vi "DMM_readout.vi"() -> ()   [LabVIEW 2009]
panel:
  out "Thermometer":dbl(slide) scale=0.0..400.0
  out "Numeric 2":i32
  in  "Samples Per Second 4":dbl=15.0
  out "CCS Resistance":dynamicdata(graph)
  out "Temperature":dbl
  out "Measurement taken":bool
  in  "stop":bool
  out "Heartbeat":bool
  in  "stop 2":bool
  out "DC coupled AC volts":string
  out "Resistance":string
  out "DC volts Chart":dbl(graph)
  out "DC volts":string
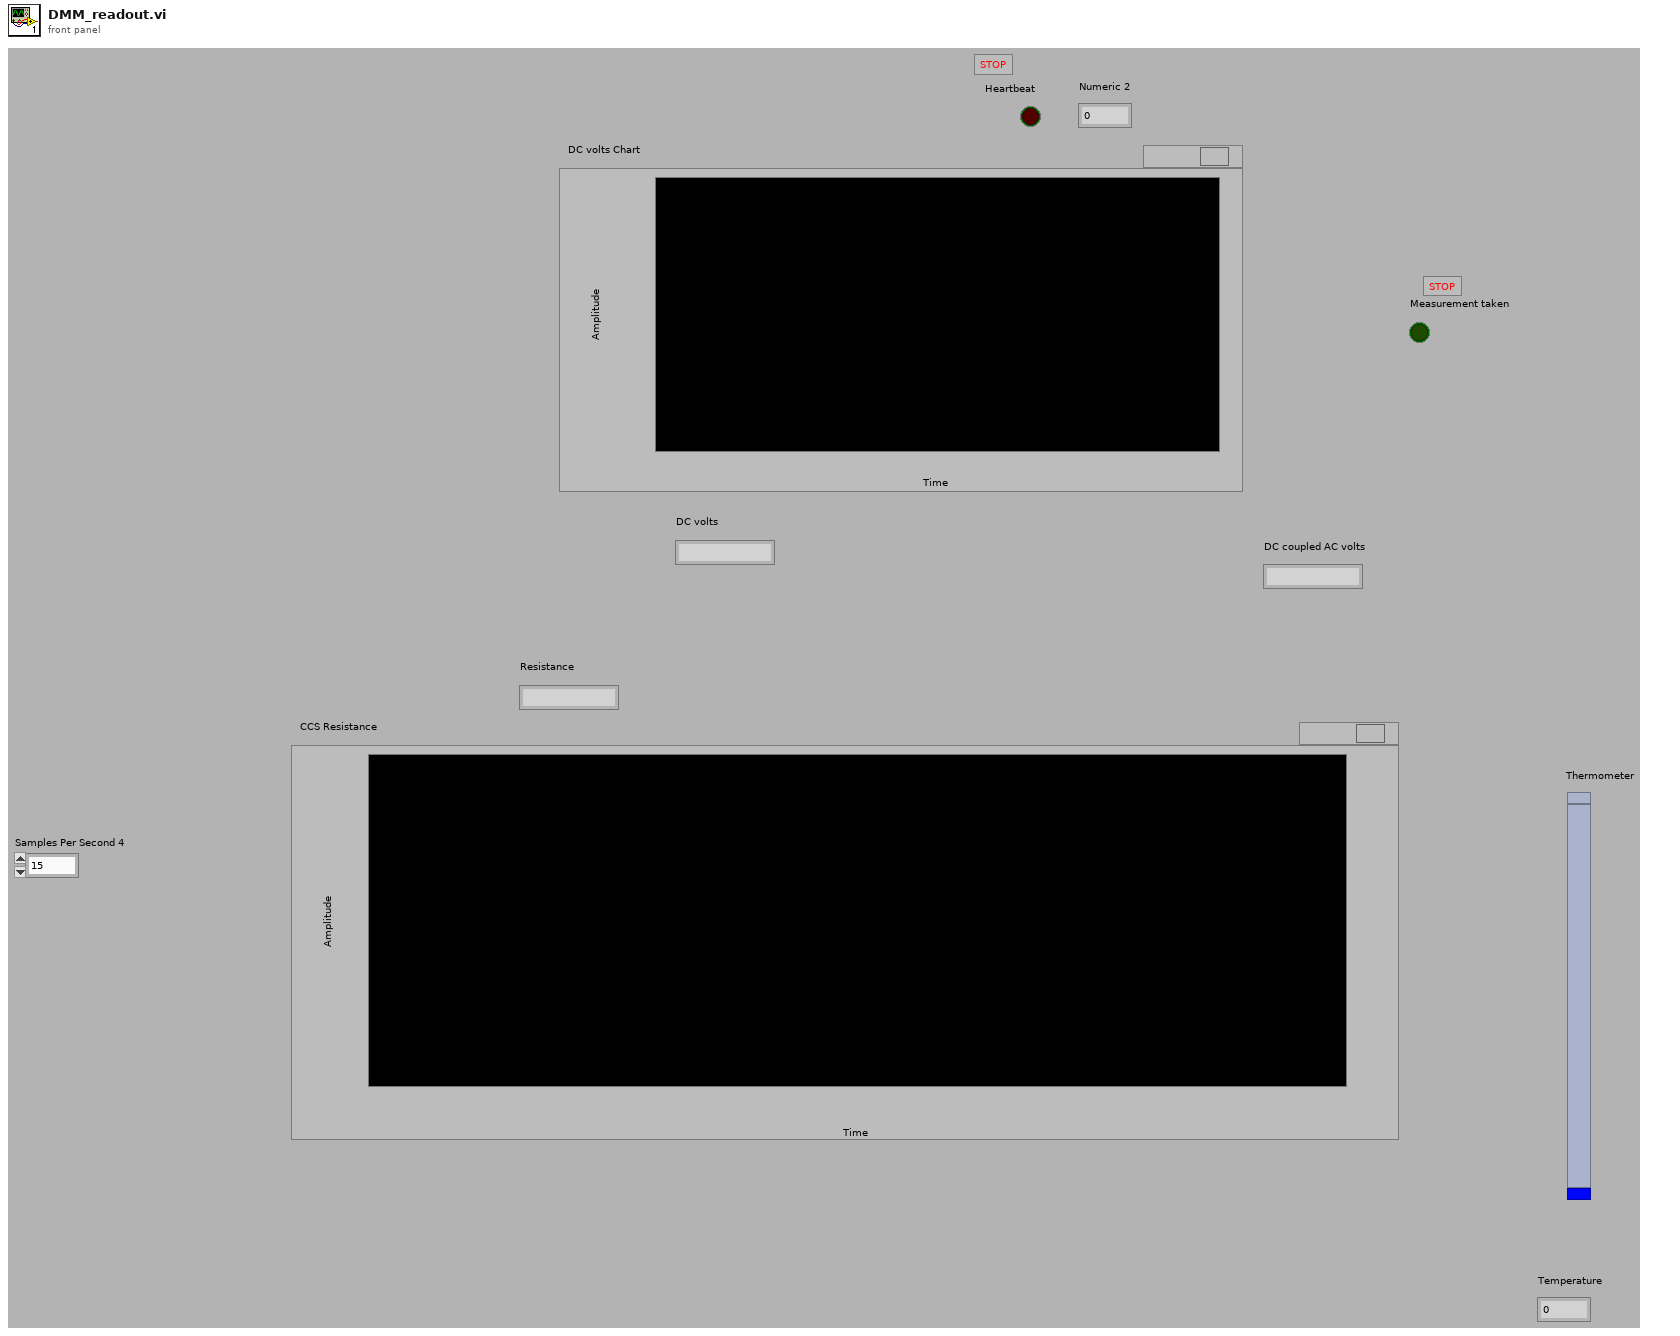
[diagram p1: front panel]
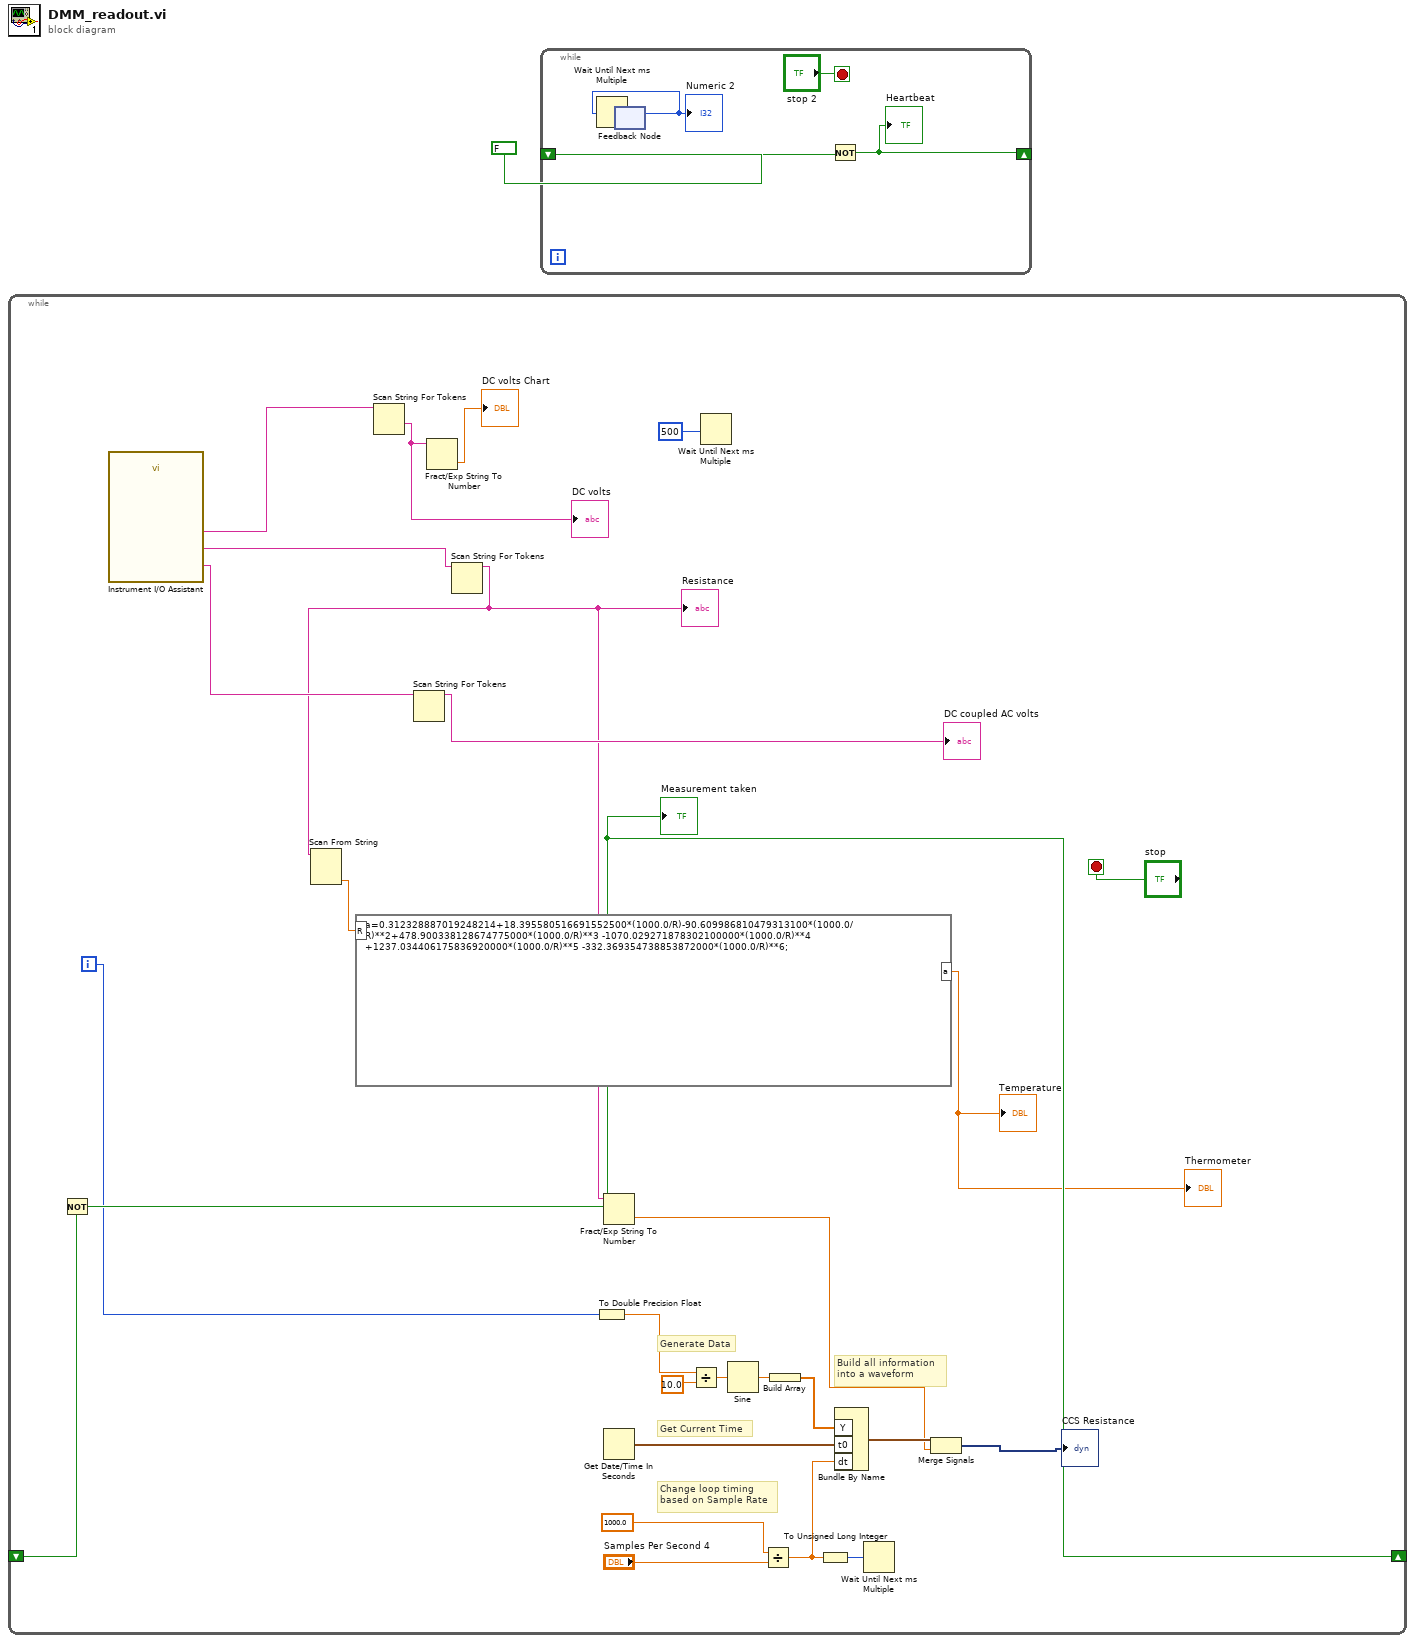
[diagram p0: block diagram]
diagram:
  n1 = while {
    shift-right: [w25] -> _
    shift-left: _ -> [w26]
    i -> [w5]
    stop <- "stop" stop-if-true
    # "Build all information\ninto a waveform"
    # "Change loop timing\nbased on Sample Rate"
    # "Get Current Time"
    # "Generate Data"
    n2 = Not(x=w26) -> (.not. x?=w25:bool)
    "Measurement taken" <- w25
    n3 = call "Instrument I/O Assistant"() -> ("DC coupled AC volts"=w20:string, "Resistance"=w18:string, "DC volts"=w23:string)  [unwired: 24 in, 1 out]
    n4 = Scan String For Tokens(9:w23) -> (1:w21:string)  [unwired: 5 in, 3 out]
    "DC volts" <- w21
    n5 = Scan String For Tokens(9:w20) -> (3:→"DC coupled AC volts":string)  [unwired: 5 in, 3 out]
    n6 = Fract/Exp String To Number(string=w21) -> (number=→"DC volts Chart":dbl)  [unwired: 3 in, 1 out]
    n7 = Scan String For Tokens(9:w18) -> (3:w17:string)  [unwired: 5 in, 3 out]
    "Resistance" <- w17
    n8 = Scan From String(input string=w17) -> (output 1=w22:dbl)  [unwired: 4 in, 3 out]
    n9 = formula code="a=0.312328887019248214+18.395580516691552500*(1000.0/R)-90.609986810479313100*(1000.0/R)**2+478.900338128674775000*(1000.0/R)**3 -1070.029271878302100000*(1000.0/R)**4 +1237.034406175836920000*(1000.0/R)**5 -332.369354738853872000*(1000.0/R)**6;"("R"=w22) -> ("a"=→"Temperature" →"Thermometer":dbl)
    n10 = To Double Precision Float(number=w5) -> (double precision float=w10:dbl)
    n11 = Fract/Exp String To Number(string=w17) -> (number=w3:dbl)  [unwired: 3 in, 1 out]
    n12 = Get Date/Time In Seconds() -> (seconds since 1Jan1904=w15:timestamp)
    n13 = Divide(x=w10, y=10.0) -> (x/y=w7:dbl)
    n14 = Wait Until Next ms Multiple(millisecond multiple=500) -> ()  [unwired: 1 out]
    n15 = Sine(x=w7) -> (sin(x)=w13:dbl)
    n16 = Divide(x=1000.0, y="Samples Per Second 4") -> (x/y=w16:dbl)
    n17 = Build Array(w13) -> (w14:dbl[])
    n18 = To Unsigned Long Integer(number=w16) -> (unsigned 32bit integer=w9:u32)
    n19 = Bundle By Name("Y"=w14, "t0"=w15, "dt"=w16) -> (w6:waveform(dbl))  [unwired: 1 in]
    n20 = Wait Until Next ms Multiple(millisecond multiple=w9) -> ()  [unwired: 1 out]
    n21 = Merge Signals(w6, w3) -> (→"CCS Resistance":dynamicdata)
  }
  n22 = while {
    shift-right: [w32] -> _
    shift-left: FALSE -> [w33]
    stop <- "stop 2" stop-if-true
    n23 = feedback #1() -> (w29:u32)  [unwired: 1 in]
    "Numeric 2" <- w29
    n24 = Wait Until Next ms Multiple(millisecond multiple=w29) -> (millisecond timer value=w30:u32)
    n25 = Not(x=w33) -> (.not. x?=w32:bool)
    "Heartbeat" <- w32
  }
